vi "Read PS Rate.vi"(8 "error in (no error)":errorcluster, 11 "PS Driver AMI4xx in":refnum<class "PS Driver AMI4xx.lvclass">) -> (0 "error out":errorcluster, 2 "Ramp rate (A/s)":dbl, 3 "PS Driver AMI4xx out":refnum<class "PS Driver AMI4xx.lvclass">)   [LabVIEW 2025, in "PS Driver.lvlib" / "PS Driver AMI4xx.lvclass"]
doc: "Author: Scott Hannahs <sth@magnet.fsu.edu>\n\nThis software is licensed for use under the “MIT License\"\nCopyright (c) 2025 Scott Hannahs, sth@sth@magnet.sthnet.net\n\nPermission is hereby granted, free of charge, to any person obtaining a copy of this software and associated documentation files (the \"Software\"), to deal in the Software without restriction, including without limitation the rights to use, copy, modify, merge, publish, distribute, sublicense, and/or sell copies of the Software, and to permit persons to whom the Software is furnished to do so, subject to the following conditions: The above copyright notice and this permission notice shall be included in all copies or substantial portions of the Software.\n\nTHE SOFTWARE IS PROVIDED \"AS IS\", WITHOUT WARRANTY OF ANY KIND, EXPRESS OR IMPLIED, INCLUDING BUT NOT LIMITED TO THE WARRANTIES OF MERCHANTABILITY, FITNESS FOR A PARTICULAR PURPOSE AND NONINFRINGEMENT. IN NO EVENT SHALL THE AUTHORS OR COPYRIGHT HOLDERS BE LIABLE FOR ANY CLAIM, DAMAGES OR OTHER LIABILITY, WHETHER IN AN ACTION OF CONTRACT, TORT OR OTHERWISE, ARISING FROM, OUT OF OR IN CONNECTION WITH THE SOFTWARE OR THE USE OR OTHER DEALINGS IN THE SOFTWARE."
uses:
  PS Driver AMI4xx.lvclass
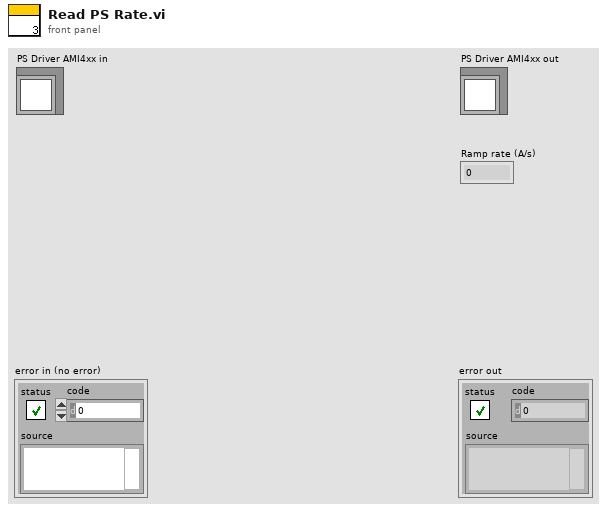
[diagram p1: front panel]
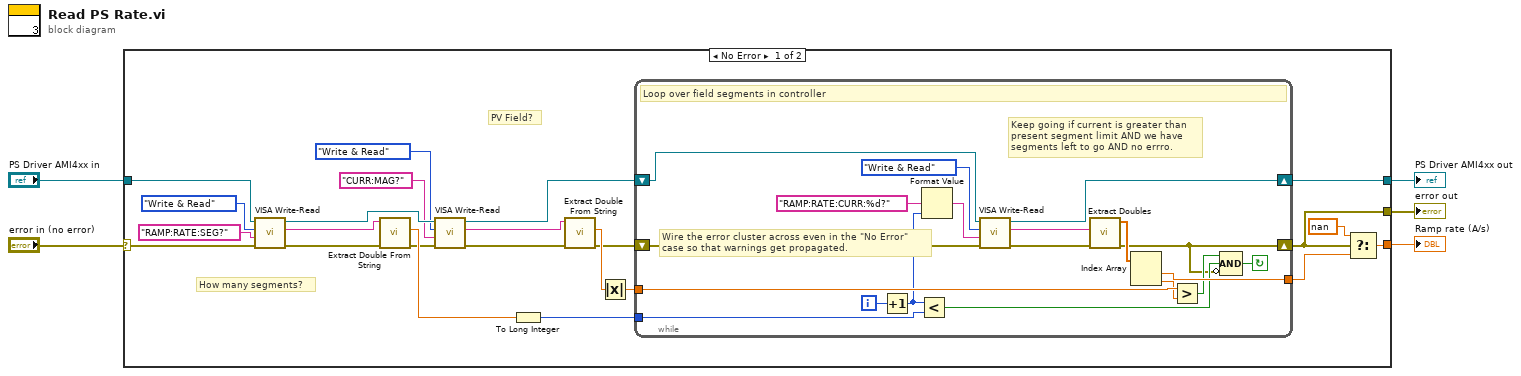
[diagram p0: block diagram]
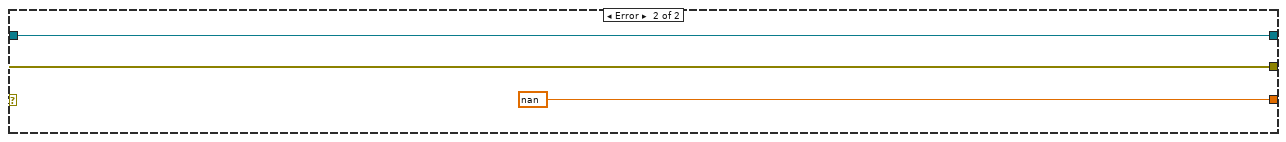
[diagram p2: hidden frame]
diagram:
  n1 = case shown="No Error" "error in (no error)" {
    selector: "error in (no error)" -> [w25 w50]
    tunnel: [w7 w50] -> w4
    tunnel: [w20 w49] -> w2
    tunnel: "PS Driver AMI4xx in" -> [w28 w49]
    tunnel: [w8 nan] -> w1
    frame No Error {
      # "PV Field?"
      # "How many segments?"
      n2 = call "VISA Write-Read.vi"("error in (no error)"=w25, "Command String"="RAMP:RATE:SEG?", "Action"=enum16{"Write", "Read", "Write & Read"}."Write & Read", "PS Driver.lvlib:PS Driver AMI4xx.lvclass"=w28) -> ("error out"=w11:errorcluster, "Response string"=w12:string, "PS Driver.lvlib:PS Driver AMI4xx.lvclass out"=w24:refnum<class "PS Driver AMI4xx.lvclass">)  [unwired: 4 in, 1 out]
      n3 = call "Extract Double From String.vi"("error in"=w11, "string"=w12) -> ("error out"=w10:errorcluster, "floating pt. number"=w13:dbl)  [unwired: 2 in, 2 out]
      n4 = call "VISA Write-Read.vi"("error in (no error)"=w10, "Command String"="CURR:MAG?", "Action"=enum16{"Write", "Read", "Write & Read"}."Write & Read", "PS Driver.lvlib:PS Driver AMI4xx.lvclass"=w24) -> ("error out"=w16:errorcluster, "Response string"=w14:string, "PS Driver.lvlib:PS Driver AMI4xx.lvclass out"=w22:refnum<class "PS Driver AMI4xx.lvclass">)  [unwired: 4 in, 1 out]
      n5 = To Long Integer(number=w13) -> (32bit integer=w9:i32)
      n6 = call "Extract Double From String.vi"("error in"=w16, "string"=w14) -> ("error out"=w15:errorcluster, "floating pt. number"=w17:dbl)  [unwired: 2 in, 2 out]
      n7 = Absolute Value(x=w17) -> (abs(x)=w21:dbl)
      n8 = while {
        shift-right: [w31] -> w20
        shift-left: w22 -> [w43]
        shift-right: [w29] -> w7
        shift-left: w15 -> [w41]
        tunnel: w21 -> [w42]
        tunnel: [w37] -> w19
        tunnel: w9 -> [w35]
        i -> [w47]
        stop <- w32 continue-if-true
        # "Wire the error cluster across even in the \"No Error\"\ncase so that warnings get propagated."
        # "Keep going if current is greater than\npresent segment limit AND we have\nsegments left to go AND no errro."
        # "Loop over field segments in controller"
        n9 = Increment(x=w47) -> (x+1=w36:i32)
        n10 = Less?(x=w36, y=w35) -> (x < y?=w33:bool)
        n11 = Format Value(format string="RAMP:RATE:CURR:%d?" ("Command String"), value (0)=w36) -> (output string=w45:string)  [unwired: 1 in]
        n12 = call "VISA Write-Read.vi"("error in (no error)"=w41, "Command String"=w45, "Action"=enum16{"Write", "Read", "Write & Read"}."Write & Read", "PS Driver.lvlib:PS Driver AMI4xx.lvclass"=w43) -> ("error out"=w30:errorcluster, "Response string"=w40:string, "PS Driver.lvlib:PS Driver AMI4xx.lvclass out"=w31:refnum<class "PS Driver AMI4xx.lvclass">)  [unwired: 4 in, 1 out]
        n13 = call "Extract Doubles.vi"("error in"=w30, "String"=w40) -> ("error out"=w29:errorcluster, "Data"=w39:dbl[])  [unwired: 4 in]
        n14 = Index Array(array=w39) -> (element #1=w37:dbl, element #2=w38:dbl)  [unwired: 2 in]
        n15 = Greater?(x=w42, y=w38) -> (0:w34:bool)
        n16 = Compound Arithmetic op=AND(w34, w33, invert w29) -> (w32:bool)
      }
      n17 = Select(t=nan, s=w7, f=w19) -> (s? t:f=w8:dbl)
    }
    frame Error {
    }
  }
  "error out" <- w4
  "PS Driver AMI4xx out" <- w2
  "Ramp rate (A/s)" <- w1
